vi "LVClass_Image Read Image.vi"(8 "error in (no error)":errorcluster, 11 "Image in":refnum<class "Image.lvclass">) -> (0 "error out":errorcluster, 2 "Image":T1, 3 "Image out":refnum<class "Image.lvclass">)   [LabVIEW 2020, in "Image.lvclass"]
uses:
  Image.lvclass
  Struct_Image.ctl
  Data alignment enum.ctl
  Point2D.ctl
  Image.lvclass/Image.ctl
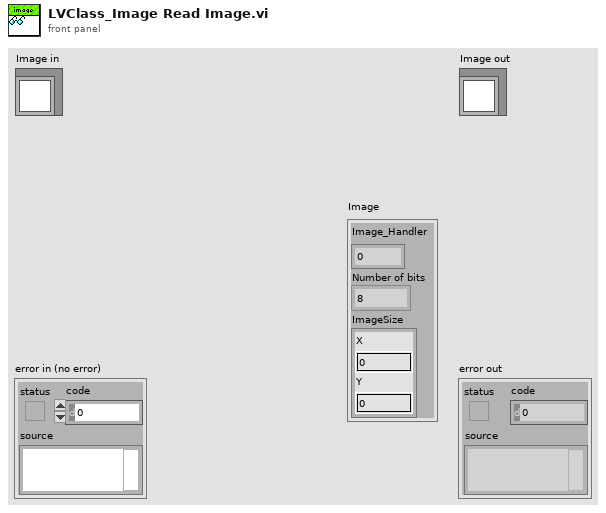
[diagram p1: front panel]
types:
  T1 = typedef "Struct_Image.ctl" = cluster{"Image_Handler":i32, "Number of bits":T2, "ImageSize":T3}
  T2 = typedef "Data alignment enum.ctl" = enum16{"8", "16", "32"}
  T3 = typedef "Point2D.ctl" = cluster{"X":u32, "Y":u32}
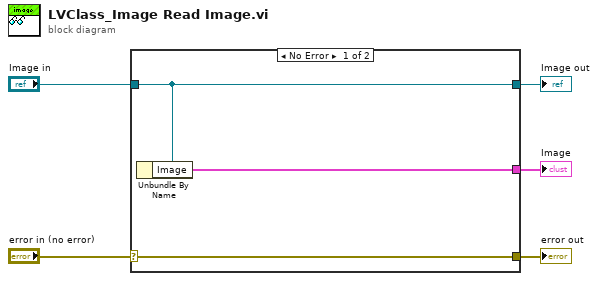
[diagram p0: block diagram]
diagram:
  n1 = case shown="No Error" "error in (no error)" {
    selector: "error in (no error)" -> [w8 w9]
    tunnel: [w8 w9] -> w4
    tunnel: [w7 w10] -> w2
    tunnel: "Image in" -> [w7 w10]
    tunnel: [w6 _] -> w1
    frame No Error {
      n2 = Unbundle By Name(w7) -> ("Image"=w6:T1)
    }
    frame Error {
    }
  }
  "error out" <- w4
  "Image out" <- w2
  "Image" <- w1
